vi "FG COP ID.vi"(1 "FG Action (Read)":T1, 2 "COP ID in":T2={"Subsystem Id"=90, "Node Id"=1, "Component Id"=1}) -> (0 "COP ID out":T2={"Subsystem Id"=90, "Node Id"=1, "Component Id"=1})   [LabVIEW 2011]
uses:
  Support Files/Address.ctl
  cRIO/Functional Global Variables/Actions for FG's.ctl
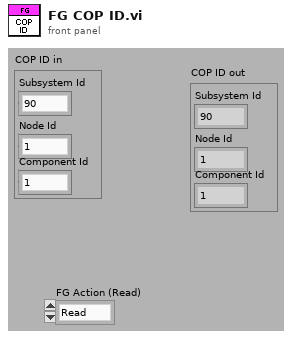
[diagram p1: front panel]
types:
  T1 = typedef "Actions for FG's.ctl" = enum16{"Read", "Write"}
  T2 = typedef "Address.ctl" = cluster{"Subsystem Id":u16, "Node Id":u8, "Component Id":u8}
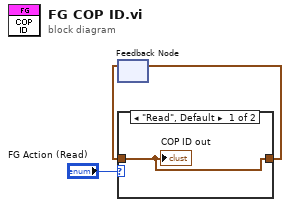
[diagram p0: block diagram]
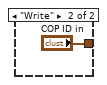
[diagram p2: hidden frame]
diagram:
  n1 = feedback #1() -> (w1:T2)  [unwired: 1 in]
  n2 = case shown="\"Read\", Default" "FG Action (Read)" {
    tunnel: w1 -> [w4 _]
    tunnel: [w4 "COP ID in"] -> w2
    frame "Read", Default {
      "COP ID out" <- w4
    }
    frame "Write" {
    }
  }
  n3 = feedback-in #1(w2) -> ()
